vi "Close.vi"(1 "DeviceHandle":i32) -> (0 "Error":bool)   [LabVIEW 2012]
uses:
  MPS-060602.dll
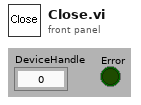
[diagram p1: front panel]
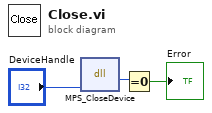
[diagram p0: block diagram]
diagram:
  n1 = dll-call lib="PTH1Yabs CDocuments and Settings\nAdministrator桌面性能\tdriver VIMPS-060602.dll" fn="MPS_CloseDevice"("DeviceHandle"="DeviceHandle") -> (w3:i32)  [unwired: 4 in, 2 out]
  n2 = Equal To 0?(x=w3) -> (x = 0?=→"Error":bool)
